vi "多参水样测试.vi"(11 "API":T1) -> ()   [LabVIEW 2016, in "HACH多参.lvlib"]
panel:
  out "结果字符串":string
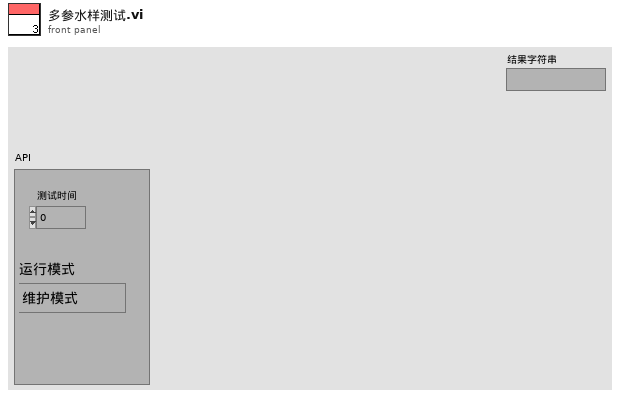
[diagram p1: front panel]
types:
  T1 = cluster{"测试时间":dbl, "运行模式":enum16{"维护模式", "常规模式", "应急模式", "质控模式"}}
  T2 = cluster{"因子编码":string, "单位":string, "水样数据时间":timestamp, "水样实测值":sgl}
  T3 = cluster{"DO_Temp":dbl, "DO_mg/L":dbl, "DO_%":dbl, "pH_Temp":dbl, "pH":dbl, "Turb":dbl, "Cond_Temp":dbl, "Cond":dbl, "Sat":dbl}
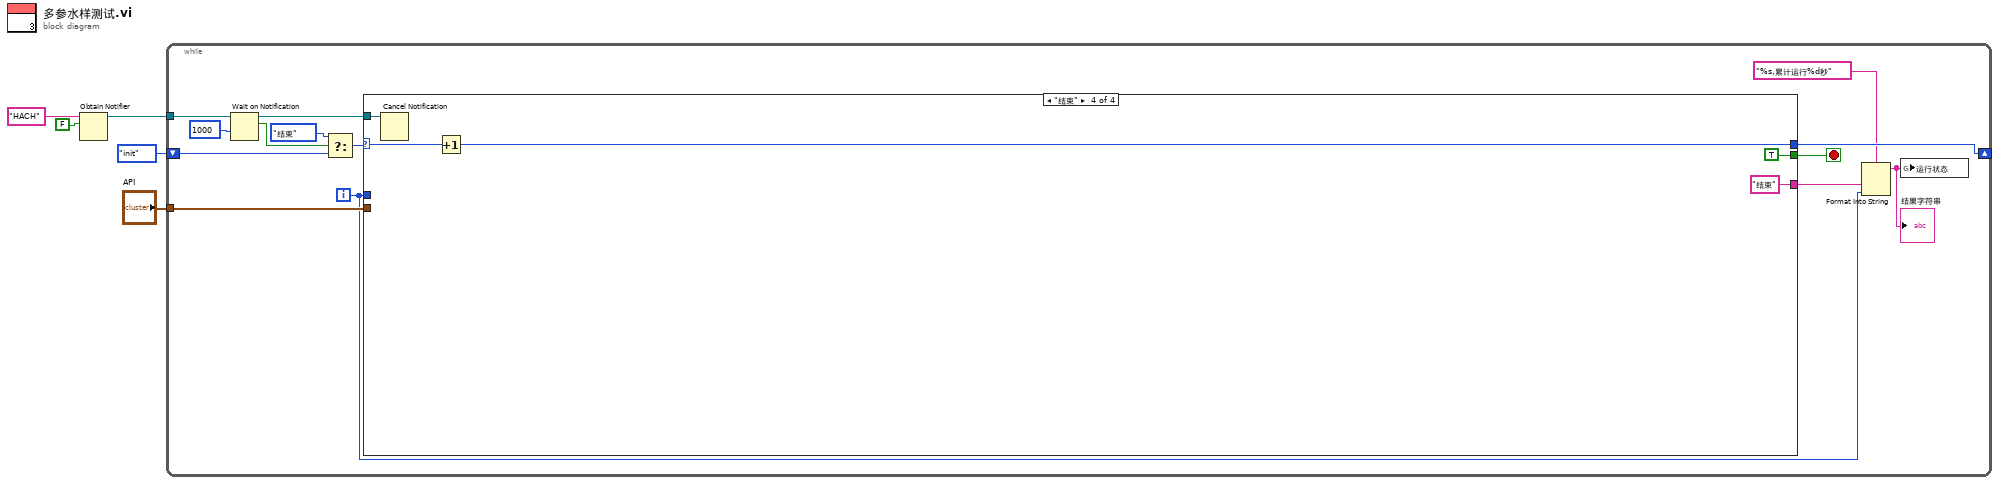
[diagram p0: block diagram]
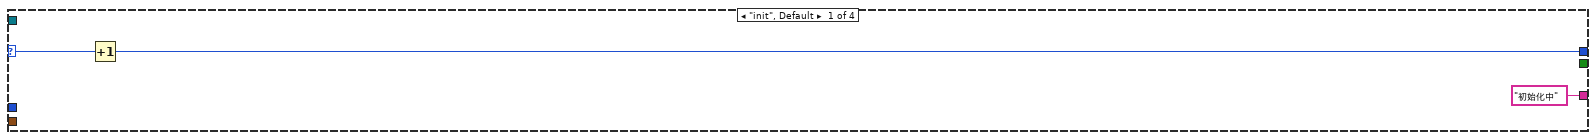
[diagram p2: hidden frame]
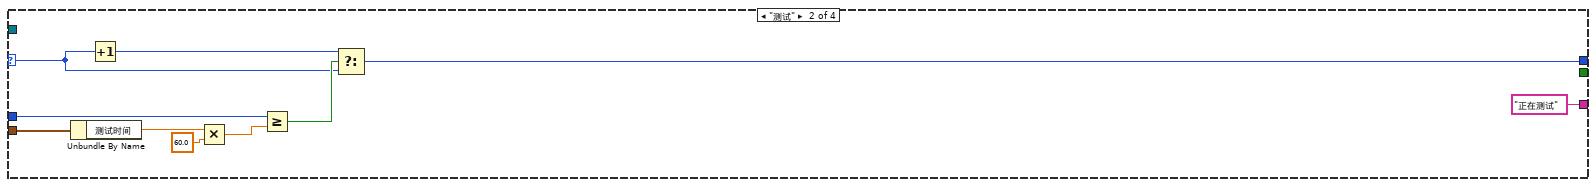
[diagram p3: hidden frame]
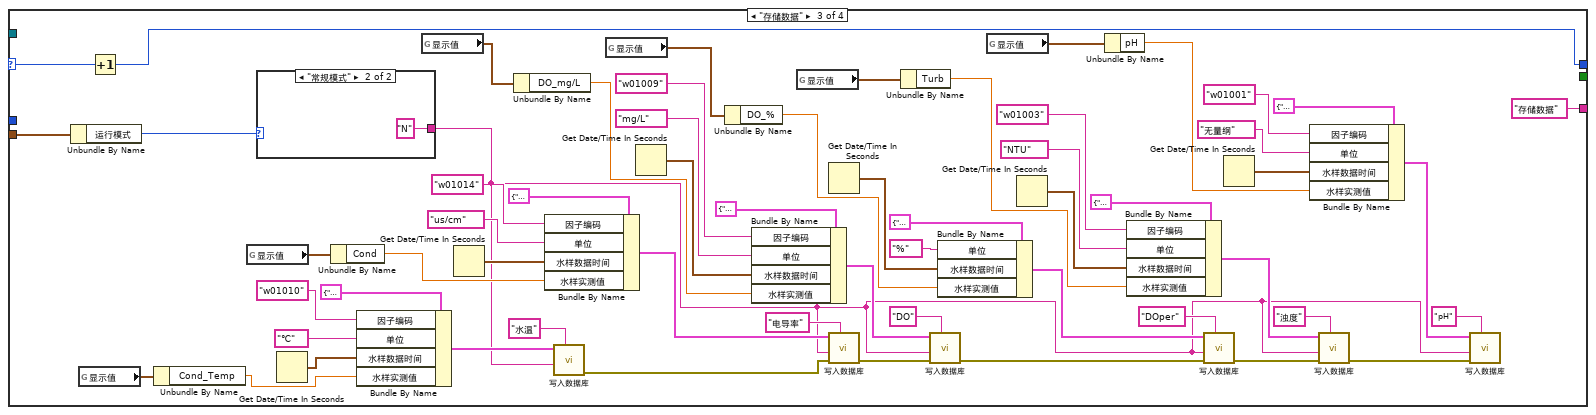
[diagram p4: hidden frame]
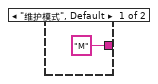
[diagram p5: hidden frame]
diagram:
  n1 = Obtain Notifier(name (unnamed)="HACH" ("名称（未命名）"), notification data type=FALSE) -> (notifier out=w1:refnum<notifier>)  [unwired: 2 in, 2 out]
  n2 = while {
    tunnel: "API" -> [w19]
    shift-right: [w18] -> _
    shift-left: enum16{"init", "测试", "存储数据", "结束"}."init" ("枚举") -> [w8]
    tunnel: w1 -> [w12]
    i -> [w14]
    stop <- w17 stop-if-true
    n3 = Wait on Notification(notifier=w12, timeout in ms (-1)=1000 ("超时毫秒(-1)")) -> (notifier out=w6:refnum<notifier>, notification=w10:bool)  [unwired: 2 in, 2 out]
    n4 = Select(t=enum16{"init", "测试", "存储数据", "结束"}."结束" ("枚举"), s=w10, f=w8) -> (s? t:f=w7:enum16{"init", "测试", "存储数据", "结束"})
    n5 = case shown="\"结束\"" w7 {
      selector: w7 -> [w22 w26 w90 w97]
      tunnel: w19 -> [_ w32 w36 _]
      tunnel: [w21 w27 w89 w96] -> w18
      tunnel: w14 -> [_ w25 _ _]
      tunnel: [_ _ _ TRUE] -> w17
      tunnel: ["初始化中" ("格式字符串") "正在测试" ("格式字符串") "存储数据" ("格式字符串") "结束" ("格式字符串")] -> w15
      tunnel: w6 -> [_ _ _ w93]
      frame "init", Default {
        n6 = Increment(x=w22) -> (x+1=w21:enum16{"init", "测试", "存储数据", "结束"})
      }
      frame "测试" {
        n7 = Unbundle By Name(w32) -> ("测试时间"=w31:dbl)
        n8 = Increment(x=w26) -> (x+1=w28:enum16{"init", "测试", "存储数据", "结束"})
        n9 = Multiply(x=w31, y=60.0) -> (x*y=w24:dbl)
        n10 = Greater Or Equal?(x=w25, y=w24) -> (x >= y?=w29:bool)
        n11 = Select(t=w28, s=w29, f=w26) -> (s? t:f=w27:enum16{"init", "测试", "存储数据", "结束"})
      }
      frame "存储数据" {
        n12 = Unbundle By Name(w36) -> ("运行模式"=w35:enum16{"维护模式", "常规模式", "应急模式", "质控模式"})
        n13 = global read "HACH全局.vi" "显示值"() -> (w48:T3)
        n14 = Increment(x=w90) -> (x+1=w89:enum16{"init", "测试", "存储数据", "结束"})
        n15 = Unbundle By Name(w48) -> ("Cond_Temp"=w47:dbl)
        n16 = global read "HACH全局.vi" "显示值"() -> (w46:T3)
        n17 = case shown="\"常规模式\"" w35 {
          tunnel: ["M" ("table输入") "N" ("table输入")] -> w34
          frame "维护模式", Default {
          }
          frame "常规模式" {
          }
        }
        n18 = Get Date/Time In Seconds() -> (seconds since 1Jan1904=w78:timestamp)
        n19 = Unbundle By Name(w46) -> ("Cond"=w45:dbl)
        n20 = Bundle By Name(cluster=T2 {"因子编码"="", "单位"="", "水样数据时间"=timestamp(0 s since 1904-01-01), "水样实测值"=0.0} ("data in"), "因子编码"="w01010", "单位"="℃", "水样数据时间"=w78, "水样实测值"=w47) -> (w50:T2)
        n21 = global read "HACH全局.vi" "显示值"() -> (w44:T3)
        n22 = Get Date/Time In Seconds() -> (seconds since 1Jan1904=w80:timestamp)
        n23 = Unbundle By Name(w44) -> ("DO_mg/L"=w43:dbl)
        n24 = Bundle By Name(cluster=T2 {"因子编码"="", "单位"="", "水样数据时间"=timestamp(0 s since 1904-01-01), "水样实测值"=0.0} ("data in"), "因子编码"="w01014", "单位"="us/cm", "水样数据时间"=w80, "水样实测值"=w45) -> (w63:T2)
        n25 = call "写入数据库.vi"("table输入"="水温", "数据标记表"=w34, "data in"=w50) -> ("error out"=w52:errorcluster)  [unwired: 8 in]
        n26 = global read "HACH全局.vi" "显示值"() -> (w42:T3)
        n27 = Get Date/Time In Seconds() -> (seconds since 1Jan1904=w82:timestamp)
        n28 = Unbundle By Name(w42) -> ("DO_%"=w41:dbl)
        n29 = Bundle By Name(cluster=T2 {"因子编码"="", "单位"="", "水样数据时间"=timestamp(0 s since 1904-01-01), "水样实测值"=0.0} ("data in"), "因子编码"="w01009", "单位"="mg/L", "水样数据时间"=w82, "水样实测值"=w43) -> (w65:T2)
        n30 = global read "HACH全局.vi" "显示值"() -> (w40:T3)
        n31 = Get Date/Time In Seconds() -> (seconds since 1Jan1904=w83:timestamp)
        n32 = call "写入数据库.vi"("table输入"="电导率", "error in (no error)"=w52, "数据标记表"=w34, "data in"=w63) -> ("error out"=w53:errorcluster)  [unwired: 7 in]
        n33 = Unbundle By Name(w40) -> ("Turb"=w39:dbl)
        n34 = call "写入数据库.vi"("table输入"="DO", "error in (no error)"=w53, "数据标记表"=w34, "data in"=w65) -> ("error out"=w54:errorcluster)  [unwired: 7 in]
        n35 = Bundle By Name(cluster=T2 {"因子编码"="", "单位"="", "水样数据时间"=timestamp(0 s since 1904-01-01), "水样实测值"=0.0} ("data in"), "单位"="%", "水样数据时间"=w83, "水样实测值"=w41) -> (w67:T2)
        n36 = global read "HACH全局.vi" "显示值"() -> (w38:T3)
        n37 = Get Date/Time In Seconds() -> (seconds since 1Jan1904=w85:timestamp)
        n38 = Unbundle By Name(w38) -> ("pH"=w37:dbl)
        n39 = Bundle By Name(cluster=T2 {"因子编码"="", "单位"="", "水样数据时间"=timestamp(0 s since 1904-01-01), "水样实测值"=0.0} ("data in"), "因子编码"="w01003", "单位"="NTU", "水样数据时间"=w85, "水样实测值"=w39) -> (w69:T2)
        n40 = call "写入数据库.vi"("table输入"="DOper", "error in (no error)"=w54, "数据标记表"=w34, "data in"=w67) -> ("error out"=w55:errorcluster)  [unwired: 7 in]
        n41 = Get Date/Time In Seconds() -> (seconds since 1Jan1904=w88:timestamp)
        n42 = Bundle By Name(cluster=T2 {"因子编码"="", "单位"="", "水样数据时间"=timestamp(0 s since 1904-01-01), "水样实测值"=0.0} ("data in"), "因子编码"="w01001", "单位"="无量纲", "水样数据时间"=w88, "水样实测值"=w37) -> (w71:T2)
        n43 = call "写入数据库.vi"("table输入"="浊度", "error in (no error)"=w55, "数据标记表"=w34, "data in"=w69) -> ("error out"=w60:errorcluster)  [unwired: 7 in]
        n44 = call "写入数据库.vi"("table输入"="pH", "error in (no error)"=w60, "数据标记表"=w34, "data in"=w71) -> ()  [unwired: 7 in, 1 out]
      }
      frame "结束" {
        n45 = Cancel Notification(0:w93) -> ()  [unwired: 1 in, 3 out]
        n46 = Increment(x=w97) -> (x+1=w96:enum16{"init", "测试", "存储数据", "结束"})
      }
    }
    n47 = Format Into String(format string="%s,累计运行%d秒" ("格式字符串"), w15, w14) -> (resulting string=w13:string)  [unwired: 2 in, 1 out]
    "结果字符串" <- w13
    n48 = global write "HACH全局.vi" "运行状态"(w13) -> ()
  }
